vi "AutoTrackRobot.vi"(11 "StartCoordinates":dbl[](array[numeric])) -> (3 "Coordinates":dbl[](array[numeric]))   [LabVIEW 2018]
uses:
  Globals.vi
  navx-mxp/labview/navX Library v2/navX Library v2.lvlib
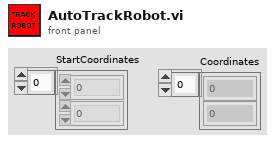
[diagram p1: front panel]
types:
  T1 = typedef "navX Library v2.lvlib/Z900_navX_DeviceTypeDef.ctl" = cluster{"Interface":cluster{"Protocol":T2, "Update Rate (4Hz-100Hz)":u8, "navX Open TypeDef":variant}, "Notify Packet":refnum<notifier>, "Loop VI Refnum":refnum<vi>, "Ready to Close Occurrence Refnum":refnum<k4>}
  T2 = typedef "navX Library v2.lvlib/Z900_navX_ProtocolTypeDef.ctl" = enum16{"SERIAL", "I2C", "SPI"}
  T3 = cluster{"Velocity X":dbl, "Velocity Y":dbl, "Velocity Z":dbl, "Displacement X":dbl, "Displacement Y":dbl, "Displacement Z":dbl}
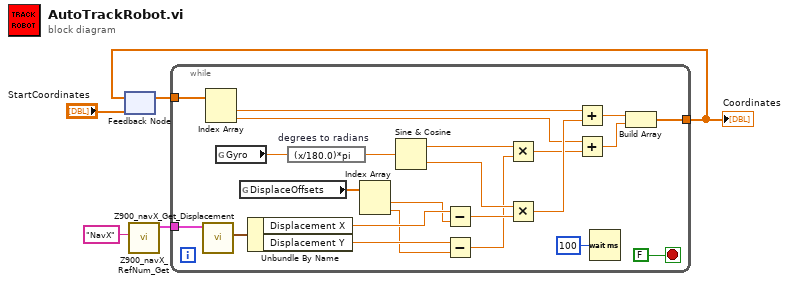
[diagram p0: block diagram]
diagram:
  n1 = feedback #1("StartCoordinates") -> (w5:dbl[])
  n2 = call "Z900_navX_RefNum_Get.vi"("refnum name"="NavX") -> ("navX Device"=w1:T1)  [unwired: 9 in, 1 out]
  n3 = while {
    tunnel: w5 -> [w26]
    tunnel: [w18] -> w3
    tunnel: w1 -> [w14]
    stop <- FALSE stop-if-true
    n4 = call "Z900_navX_Get_Displacement.vi"("navX Device"=w14) -> ("Displacement"=w15:T3)  [unwired: 7 in, 3 out]
    n5 = Index Array(array=w26) -> (element #1=w25:dbl, element #2=w22:dbl)  [unwired: 2 in]
    n6 = global read "Globals.vi" "Gyro"() -> (w27:dbl)
    n7 = global read "Globals.vi" "DisplaceOffsets"() -> (w12:dbl[])
    n8 = Unbundle By Name(w15) -> ("Displacement X"=w9:dbl, "Displacement Y"=w10:dbl)
    n9 = expression code="(x/180.0)*pi" "degrees to radians"(w27) -> (w16:dbl)
    n10 = Index Array(array=w12) -> (element #1=w8:dbl, element #2=w7:dbl)  [unwired: 2 in]
    n11 = Sine & Cosine(0:w16) -> (1:w24:dbl, 2:w13:dbl)
    n12 = Subtract(x=w9, y=w8) -> (x-y=w11:dbl)
    n13 = Subtract(x=w10, y=w7) -> (x-y=w6:dbl)
    n14 = Multiply(x=w24, y=w6) -> (x*y=w21:dbl)
    n15 = Multiply(x=w13, y=w11) -> (x*y=w23:dbl)
    n16 = Add(x=w25, y=w23) -> (x+y=w20:dbl)
    n17 = Add(x=w22, y=w21) -> (x+y=w19:dbl)
    n18 = Wait (ms)(milliseconds to wait=u32 100) -> ()  [unwired: 1 out]
    n19 = Build Array(w20, w19) -> (w18:dbl[])
  }
  "Coordinates" <- w3
  n20 = feedback-in #1(w3) -> ()
